vi "5x PNS lesen.vi"(8 "Fehler (Eingang, kein Fehler)":errorcluster, 9 "IP Adresse":string, 10 "Grenzwerte PNS (Eingang)":T1 {"Heizleitung 6:"."Regler" items=["aktiv", "inaktiv"]; "Heizleitung 6:"."Abschalt-Max" format="%#_5g"; "Heizleitung 6:"."Abschalt-Min" format="%#_5g"; "Heizleitung 6:"."Warn-Max" format="%#_5g"; "Heizleitung 6:"."Warn-Min" format="%#_5g"; "Heizleitung 6:"."Sollwert" format="%#_5g"; "Heizleitung 5:"."Regler" items=["aktiv", "inaktiv"]; "Heizleitung 5:"."Abschalt-Max" format="%#_5g"; "Heizleitung 5:"."Abschalt-Min" format="%#_5g"; "Heizleitung 5:"."Warn-Max" format="%#_5g"; "Heizleitung 5:"."Warn-Min" format="%#_5g"; "Heizleitung 5:"."Sollwert" format="%#_5g"; "Heizleitung 4:"."Regler" items=["aktiv", "inaktiv"]; "Heizleitung 4:"."Abschalt-Max" format="%#_5g"; "Heizleitung 4:"."Abschalt-Min" format="%#_5g"; "Heizleitung 4:"."Warn-Max" format="%#_5g"; "Heizleitung 4:"."Warn-Min" format="%#_5g"; "Heizleitung 4:"."Sollwert" format="%#_5g"; "Heizleitung 3:"."Regler" items=["aktiv", "inaktiv"]; "Heizleitung 3:"."Abschalt-Max" format="%#_5g"; "Heizleitung 3:"."Abschalt-Min" format="%#_5g"; "Heizleitung 3:"."Warn-Max" format="%#_5g"; "Heizleitung 3:"."Warn-Min" format="%#_5g"; "Heizleitung 3:"."Sollwert" format="%#_5g"; "Heizleitung 2:"."Regler" items=["aktiv", "inaktiv"]; "Heizleitung 2:"."Abschalt-Max" format="%#_5g"; "Heizleitung 2:"."Abschalt-Min" format="%#_5g"; "Heizleitung 2:"."Warn-Max" format="%#_5g"; "Heizleitung 2:"."Warn-Min" format="%#_5g"; "Heizleitung 2:"."Sollwert" format="%#_5g"; "Heizleitung 1:"."Regler" items=["aktiv", "inaktiv"]; "Heizleitung 1:"."Abschalt-Max" format="%#_5g"; "Heizleitung 1:"."Abschalt-Min" format="%#_5g"; "Heizleitung 1:"."Warn-Max" format="%#_5g"; "Heizleitung 1:"."Warn-Min" format="%#_5g"; "Heizleitung 1:"."Sollwert" format="%#_5g"; "Ventilplatte:"."Regler" items=["aktiv", "inaktiv"]; "Ventilplatte:"."Abschalt-Max" format="%#_5g"; "Ventilplatte:"."Abschalt-Min" format="%#_5g"; "Ventilplatte:"."Warn-Max" format="%#_5g"; "Ventilplatte:"."Warn-Min" format="%#_5g"; "Ventilplatte:"."Sollwert" format="%#_5g"; "Filter:"."Regler" items=["aktiv", "inaktiv"]; "Filter:"."Abschalt-Max" format="%#_5g"; "Filter:"."Abschalt-Min" format="%#_5g"; "Filter:"."Warn-Max" format="%#_5g"; "Filter:"."Warn-Min" format="%#_5g"; "Filter:"."Sollwert" format="%#_5g"}, 11 "Dateipfad im Ordner des Haupt-VIs":path) -> (0 "Fehler (Ausgang)":errorcluster, 2 "IP Adresse":string, 3 "Grenzwerte PNS (Ausgang)":T1 {"Heizleitung 6:"."Regler" items=["aktiv", "inaktiv"]; "Heizleitung 6:"."Abschalt-Max" format="%#_5g"; "Heizleitung 6:"."Abschalt-Min" format="%#_5g"; "Heizleitung 6:"."Warn-Max" format="%#_5g"; "Heizleitung 6:"."Warn-Min" format="%#_5g"; "Heizleitung 6:"."Sollwert" format="%#_5g"; "Heizleitung 5:"."Regler" items=["aktiv", "inaktiv"]; "Heizleitung 5:"."Abschalt-Max" format="%#_5g"; "Heizleitung 5:"."Abschalt-Min" format="%#_5g"; "Heizleitung 5:"."Warn-Max" format="%#_5g"; "Heizleitung 5:"."Warn-Min" format="%#_5g"; "Heizleitung 5:"."Sollwert" format="%#_5g"; "Heizleitung 4:"."Regler" items=["aktiv", "inaktiv"]; "Heizleitung 4:"."Abschalt-Max" format="%#_5g"; "Heizleitung 4:"."Abschalt-Min" format="%#_5g"; "Heizleitung 4:"."Warn-Max" format="%#_5g"; "Heizleitung 4:"."Warn-Min" format="%#_5g"; "Heizleitung 4:"."Sollwert" format="%#_5g"; "Heizleitung 3:"."Regler" items=["aktiv", "inaktiv"]; "Heizleitung 3:"."Abschalt-Max" format="%#_5g"; "Heizleitung 3:"."Abschalt-Min" format="%#_5g"; "Heizleitung 3:"."Warn-Max" format="%#_5g"; "Heizleitung 3:"."Warn-Min" format="%#_5g"; "Heizleitung 3:"."Sollwert" format="%#_5g"; "Heizleitung 2:"."Regler" items=["aktiv", "inaktiv"]; "Heizleitung 2:"."Abschalt-Max" format="%#_5g"; "Heizleitung 2:"."Abschalt-Min" format="%#_5g"; "Heizleitung 2:"."Warn-Max" format="%#_5g"; "Heizleitung 2:"."Warn-Min" format="%#_5g"; "Heizleitung 2:"."Sollwert" format="%#_5g"; "Heizleitung 1:"."Regler" items=["aktiv", "inaktiv"]; "Heizleitung 1:"."Abschalt-Max" format="%#_5g"; "Heizleitung 1:"."Abschalt-Min" format="%#_5g"; "Heizleitung 1:"."Warn-Max" format="%#_5g"; "Heizleitung 1:"."Warn-Min" format="%#_5g"; "Heizleitung 1:"."Sollwert" format="%#_5g"; "Ventilplatte:"."Regler" items=["aktiv", "inaktiv"]; "Ventilplatte:"."Abschalt-Max" format="%#_5g"; "Ventilplatte:"."Abschalt-Min" format="%#_5g"; "Ventilplatte:"."Warn-Max" format="%#_5g"; "Ventilplatte:"."Warn-Min" format="%#_5g"; "Ventilplatte:"."Sollwert" format="%#_5g"; "Filter:"."Regler" items=["aktiv", "inaktiv"]; "Filter:"."Abschalt-Max" format="%#_5g"; "Filter:"."Abschalt-Min" format="%#_5g"; "Filter:"."Warn-Max" format="%#_5g"; "Filter:"."Warn-Min" format="%#_5g"; "Filter:"."Sollwert" format="%#_5g"})   [LabVIEW 2015, in "allgemeine Sub-VIs.lvlib"]
uses:
  allgemeine Sub-VIs.lvlib
  PNS/Anlagengrenzwerte PNS.ctl
  PNS/Anlagengrenzwerte-Parameter Anzeige.ctl
  Visualisierungs Elemente/Zahlen-Eingabefeld.ctl
  PNS/PNS.lvlib
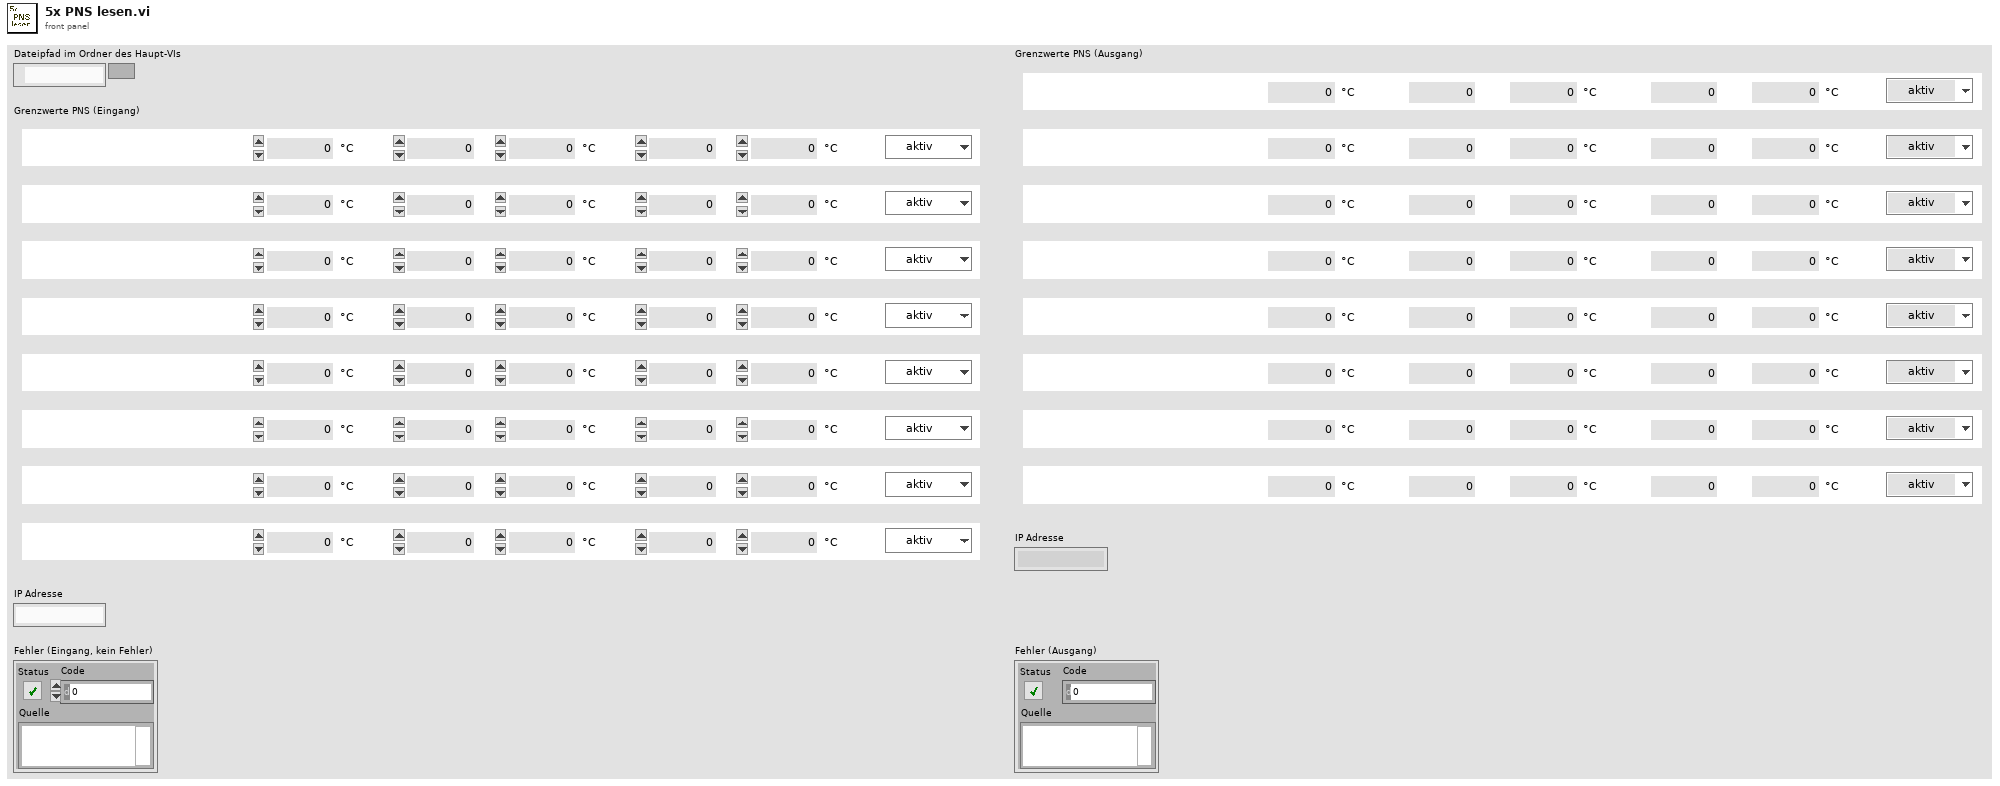
[diagram p1: front panel]
types:
  T1 = typedef "PNS.lvlib/Anlagengrenzwerte PNS.ctl" = cluster{"Filter:":T2, "Ventilplatte:":T2, "Heizleitung 1:":T2, "Heizleitung 2:":T2, "Heizleitung 3:":T2, "Heizleitung 4:":T2, "Heizleitung 5:":T2, "Heizleitung 6:":T2}
  T2 = typedef "PNS.lvlib/Anlagengrenzwerte-Parameter Anzeige.ctl" = cluster{"Sollwert":T3, "Warn-Min":T3, "Warn-Max":T3, "Abschalt-Min":T3, "Abschalt-Max":T3, "Regler":u16, "AnlagenParameter":string}
  T3 = typedef "Zahlen-Eingabefeld.ctl" = sgl
  T4 = cluster{"Grenzwerte PNS (Eingang)":T1, "IP Adresse":string}
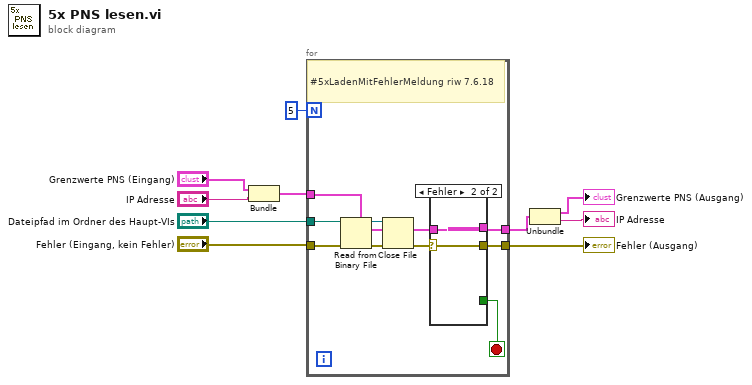
[diagram p0: block diagram]
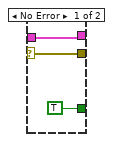
[diagram p2: hidden frame]
diagram:
  n1 = Bundle("Grenzwerte PNS (Eingang)"="Grenzwerte PNS (Eingang)", "IP Adresse"="IP Adresse") -> (w6:T4)  [unwired: 1 in]
  n2 = for {
    N: 5 -> [_]
    tunnel: "Dateipfad im Ordner des Haupt-VIs" -> [w18]
    tunnel: "Fehler (Eingang, kein Fehler)" -> [w20]
    tunnel: [w17] -> w10
    tunnel: w6 -> [w19]
    tunnel: [w15] -> w1
    stop <- w14 stop-if-true
    # "#5xLadenMitFehlerMeldung riw 7.6.18"
    n3 = Read from Binary File(5:w19, 8:w20, 11:w18) -> (0:w12:errorcluster, 2:w16:T4, 3:w13:refnum<file>)  [unwired: 4 out]
    n4 = Close File(refnum=w13, error in=w12) -> (error out=w11:errorcluster)  [unwired: 1 out]
    n5 = case shown="Fehler" w11 {
      selector: w11 -> [w23 w25]
      tunnel: [w23 w25] -> w17
      tunnel: w16 -> [w22 w24]
      tunnel: [w22 w24] -> w15
      tunnel: [TRUE _] -> w14
      frame No Error {
      }
      frame Error {
      }
    }
  }
  "Fehler (Ausgang)" <- w10
  n6 = Unbundle(w1) -> ("Grenzwerte PNS (Eingang)"=→"Grenzwerte PNS (Ausgang)":T1, "IP Adresse"=→"IP Adresse":string)
